vi "Trial v2.vi"(2 "error in (no error)":errorcluster, 3 "queue in":refnum<queue>, 4 "DDA":bool=TRUE) -> (0 "error out":errorcluster, 1 "queue out":refnum<queue>)   [LabVIEW 2017]
uses:
  SubVI/Global.vi
  <vilib>/Analysis/NI_AALPro.lvlib
  <vilib>/robotics/Kinematics/NI_Kinematics.lvlib
  Control/RPY.ctl
  Control/Damping.ctl
  <vilib>/Analysis/NI_AALBase.lvlib
  <vilib>/Analysis/baseanly.llb/Real Dot Product.vi
  <vilib>/Analysis/_algsub.llb/Real Vector Norm.vi
panel:
  in  "Algorithm Parameter":T1={"lambda w"=0.99, "lambda theta"=0.99, "alpha w"=0.01, "alpha theta"=0.01, "alpha Rbar"=0.01}
  in  "n":i32=2
  in  "Reward Parameter":cluster{"C":dbl, "alpha":dbl}={"C"=10.0, "alpha"=1.0}
  in  "lower limit (RoM)":dbl=15.0
  in  "upper limit (RoM)":dbl=85.0
  in  "Time Target (s)":dbl=5.0
  in  "epsilon":dbl=0.1
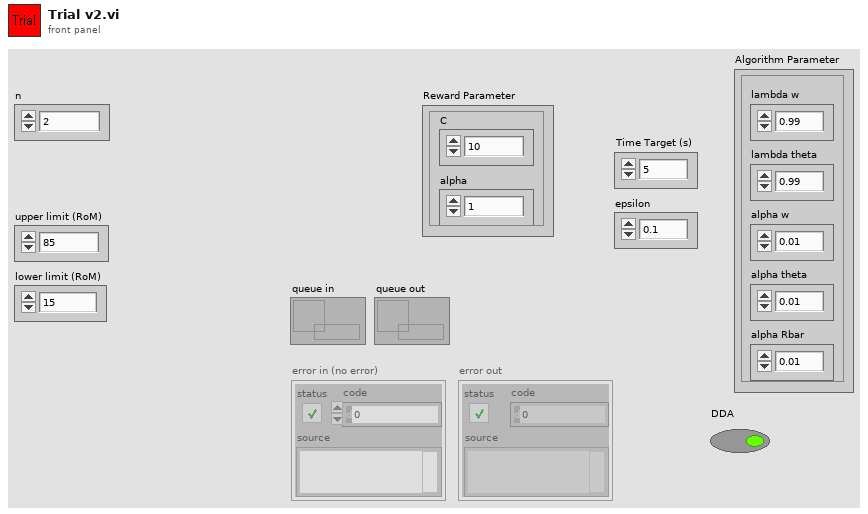
[diagram p1: front panel]
types:
  T1 = cluster{"lambda w":dbl, "lambda theta":dbl, "alpha w":dbl, "alpha theta":dbl, "alpha Rbar":dbl}
  T2 = typedef "Damping.ctl" = cluster{"Cx":dbl, "Cy":dbl, "Cz":dbl}
  T3 = typedef "RPY.ctl" = cluster{"roll":dbl, "pitch":dbl, "yaw":dbl}
  T4 = typedef "NI_Matrix.lvlib/RealMatrix.ctl" = dbl[][]
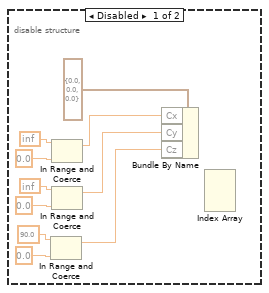
[diagram p2: hidden frame]
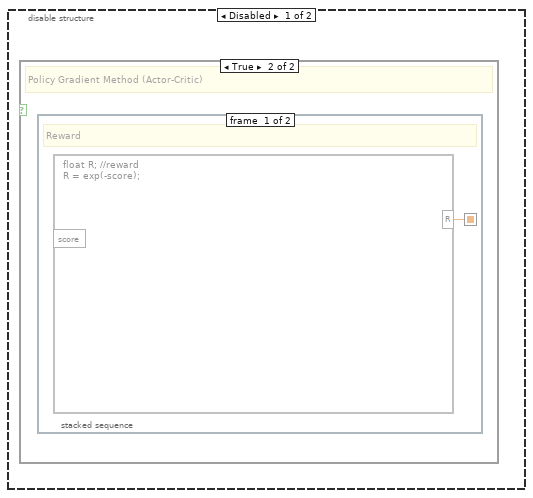
[diagram p3: hidden frame]
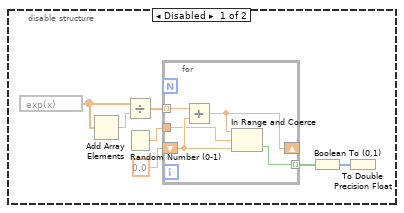
[diagram p6: hidden frame]
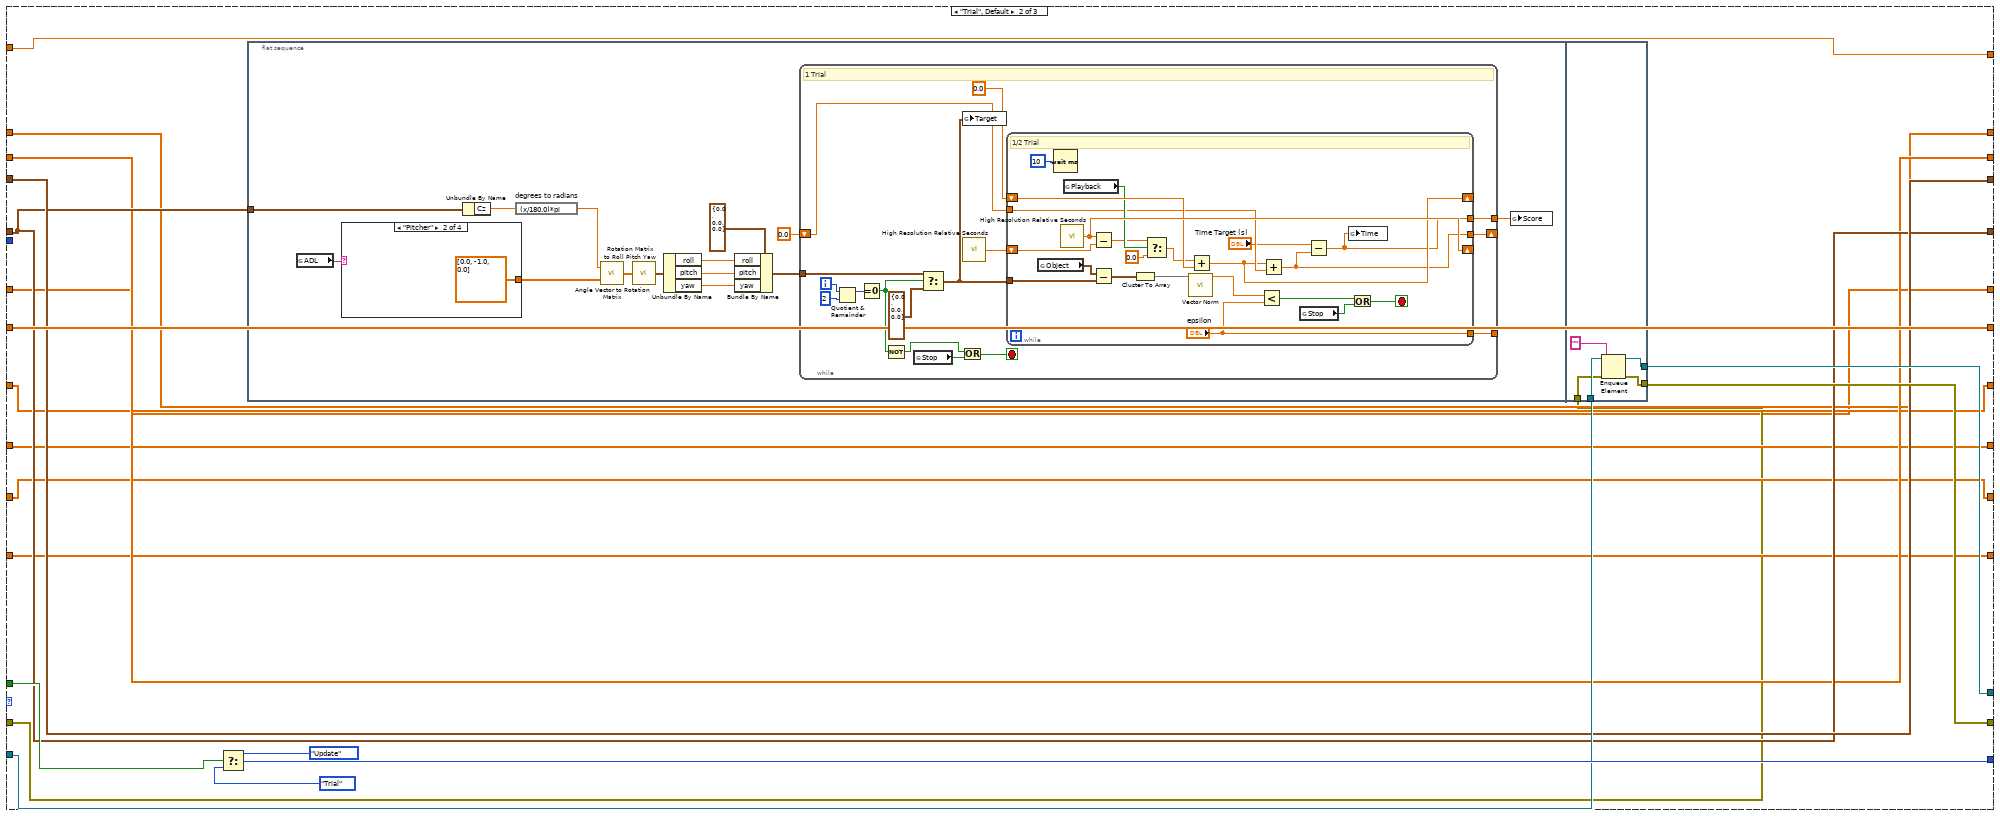
[diagram p7: hidden frame]
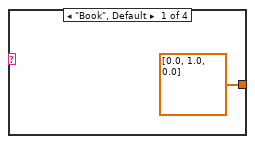
[diagram p8: hidden frame]
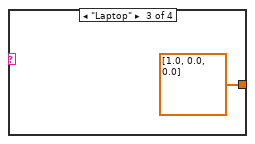
[diagram p9: hidden frame]
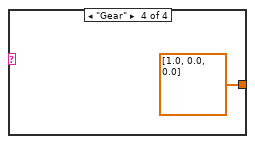
[diagram p10: hidden frame]
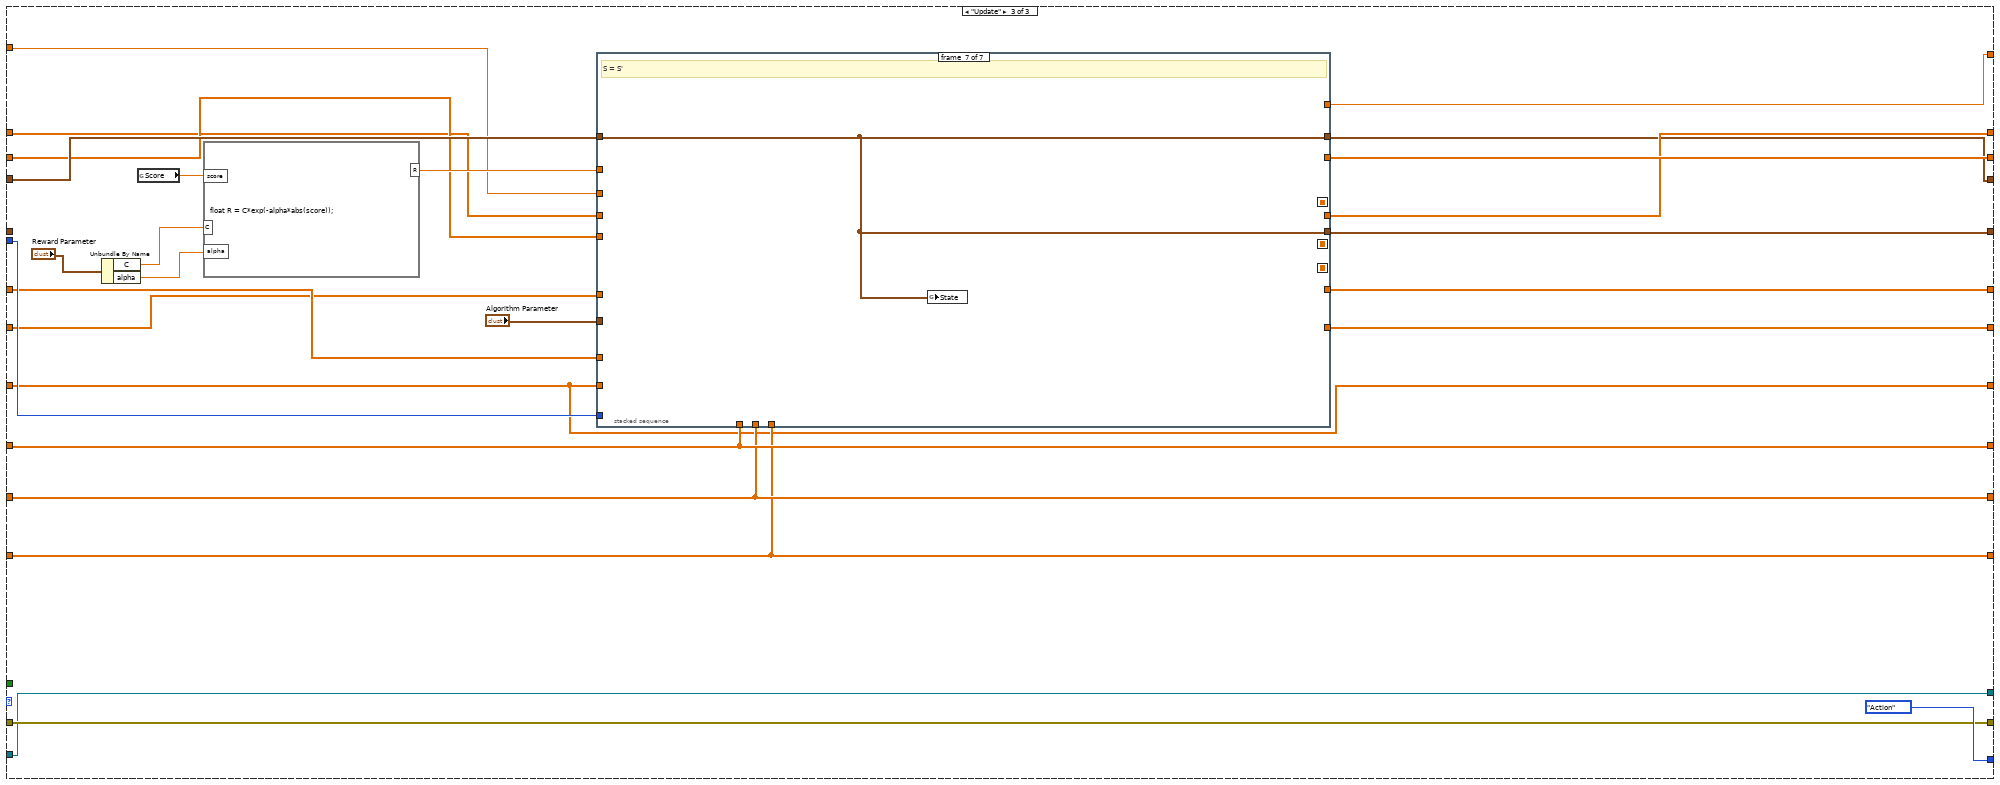
[diagram p11: hidden frame]
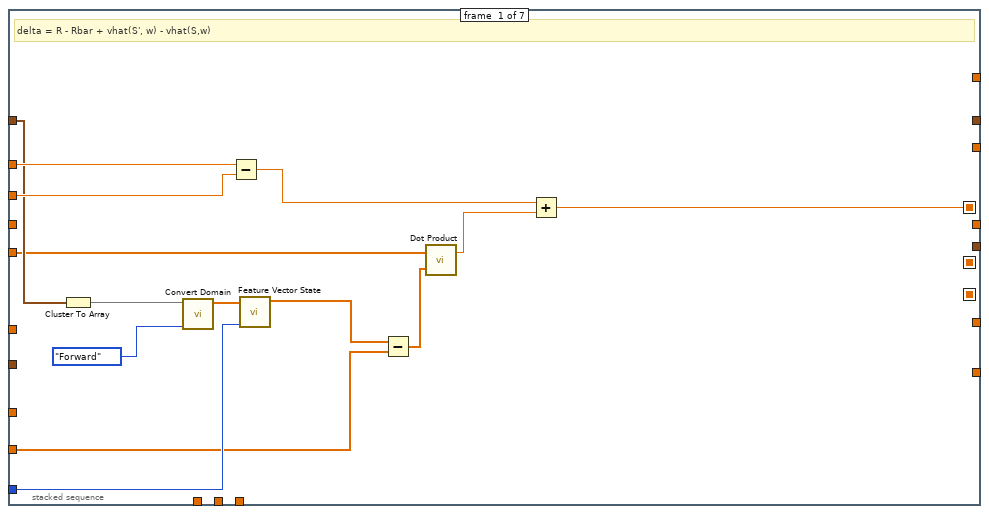
[diagram p12: hidden frame]
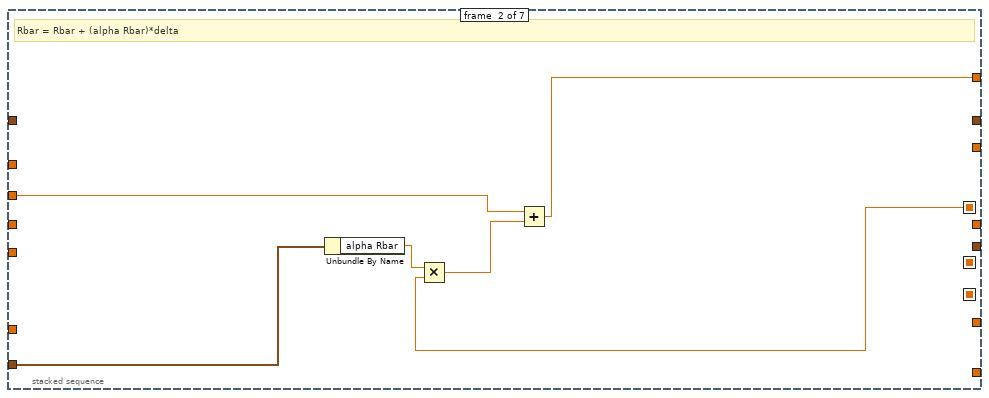
[diagram p13: hidden frame]
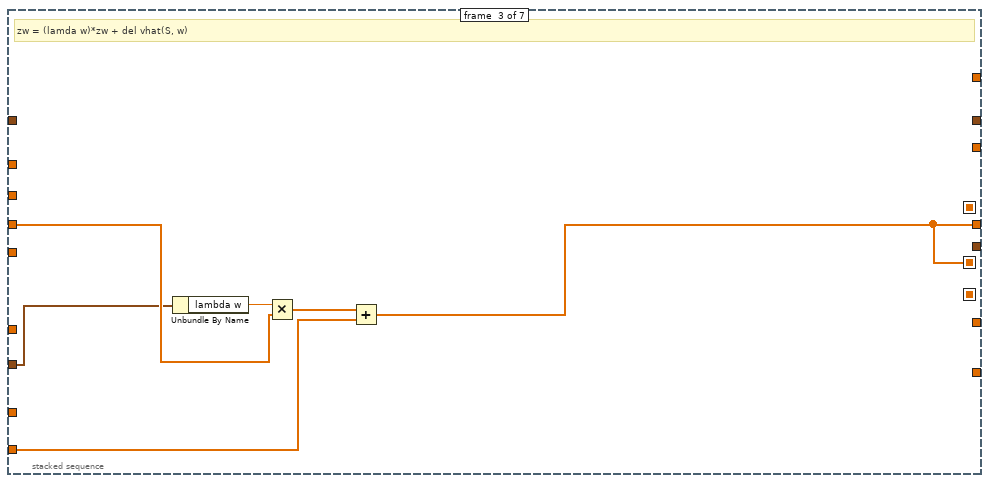
[diagram p14: hidden frame]
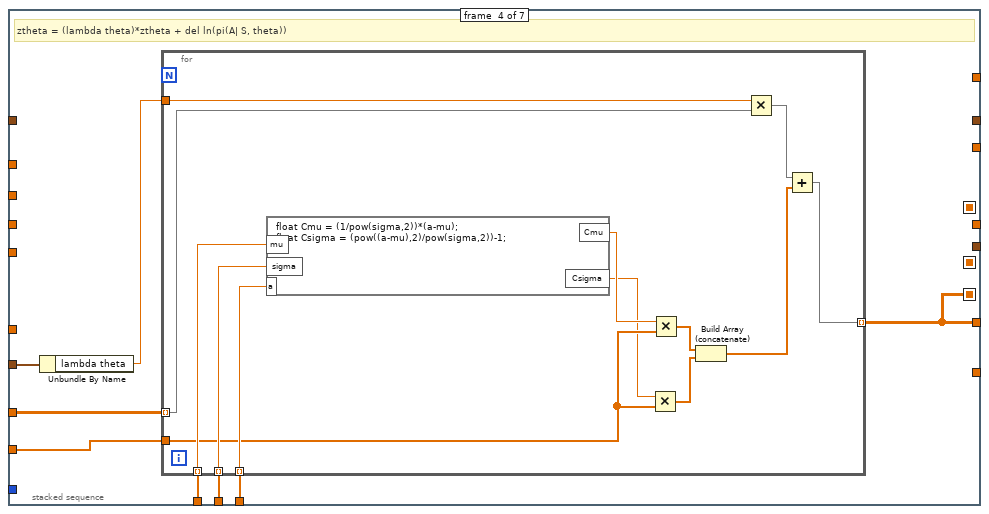
[diagram p15: hidden frame]
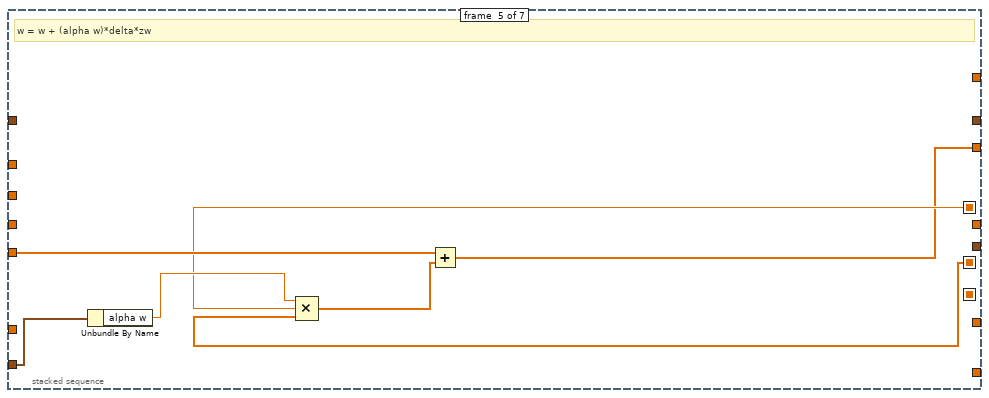
[diagram p16: hidden frame]
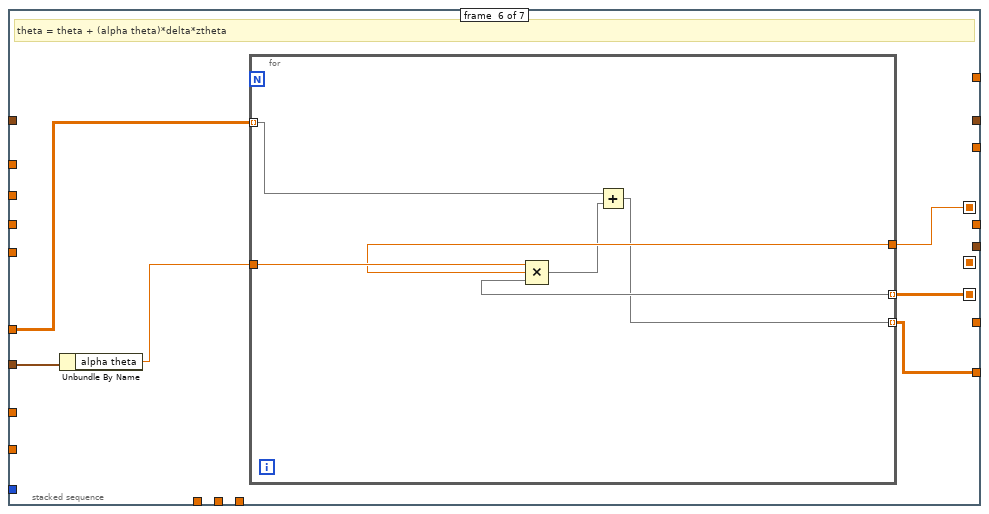
[diagram p17: hidden frame]
diagram:
  n1 = flat-sequence {
    tunnel: "error in (no error)" -> [w23]
    tunnel: "queue in" -> [w25]
    tunnel: "DDA" -> [w18]
    tunnel: [w24] -> w2
    tunnel: [w22] -> w1
    frame #0 {
      n2 = flat-sequence {
        tunnel: ["n"] -> w17
        tunnel: [w38] -> w16
        tunnel: [w37] -> w15
        tunnel: [w37] -> w14
        tunnel: [w31] -> w13
        tunnel: [w29] -> w12
        tunnel: [w29] -> w11
        tunnel: [w31] -> w10
        tunnel: [w29] -> w9
        tunnel: [dbl[] [0.0, 0.0, 0.0]] -> w8
        tunnel: [dbl[] [1.0, 1.0, 1.0]] -> w7
        tunnel: [dbl[] [0.0, 0.0, 0.0]] -> w6
        frame #0 {
          w38 = 0.0  # Rbar
          n3 = call "Feature Vector State.vi"("n x(s)"="n", "state"=dbl[] [0.0, 0.0, 0.0] ("array")) -> ("x(s)"=w34:dbl[])  [unwired: 9 in]
          n4 = Array Size(array=w34) -> (size(s)=w33:i32)
          n5 = Initialize Array(0.0, w33) -> (w29:dbl[])
          n6 = global read "Global.vi" "State"() -> (w37:T2)
          n7 = Build Array (concatenate)(w29, w29) -> (w36:dbl[])
          n8 = Build Array(w36, w36, w36) -> (w31:dbl[][])
        }
      }
      n9 = Select(t=enum16{"Action", "Trial", "Update"}."Action", s=w18, f=enum16{"Action", "Trial", "Update"}."Trial") -> (s? t:f=w19:enum16{"Action", "Trial", "Update"})
      n10 = while {
        shift-right: [w63] -> w24
        shift-left: w25 -> [w65]
        shift-right: [w62] -> w22
        shift-left: w23 -> [w64]
        shift-right: [w67] -> _
        shift-left: w19 -> [w68]
        tunnel: w18 -> [w66]
        tunnel: w17 -> [w61]
        shift-right: [w60] -> _
        shift-left: w13 -> [w59]
        shift-right: [w57] -> _
        shift-left: w16 -> [w58]
        shift-right: [w53] -> _
        shift-left: w15 -> [w55]
        shift-right: [w56] -> _
        shift-left: w14 -> [w54]
        shift-right: [w51] -> _
        shift-left: w12 -> [w52]
        shift-right: [w49] -> _
        shift-left: w11 -> [w50]
        shift-right: [w39] -> _
        shift-left: w10 -> [w48]
        shift-right: [w47] -> _
        shift-left: w9 -> [w46]
        shift-right: [w45] -> _
        shift-left: w8 -> [w44]
        shift-right: [w42] -> _
        shift-left: w7 -> [w43]
        shift-right: [w40] -> _
        shift-left: w6 -> [w41]
        stop <- w69 stop-if-true
        # "State Machine"
        n11 = case shown="\"Action\"" w68 {
          tunnel: [enum16{"Action", "Trial", "Update"}."Trial" w129 enum16{"Action", "Trial", "Update"}."Action"] -> w67
          tunnel: w66 -> [_ w131 _]
          tunnel: w65 -> [w84 w128 w217]
          tunnel: w64 -> [w85 w114 w218]
          tunnel: [w84 w127 w217] -> w63
          tunnel: [w85 w126 w218] -> w62
          tunnel: w61 -> [w77 _ w208]
          tunnel: [w83 w124 w196] -> w60
          tunnel: w59 -> [w83 w124 w198]
          tunnel: w58 -> [w80 w123 w210]
          tunnel: [w80 w123 w206] -> w57
          tunnel: w55 -> [w78 w121 _]
          tunnel: [w79 w122 w195] -> w56
          tunnel: w54 -> [_ w122 w212]
          tunnel: [w78 w121 w194] -> w53
          tunnel: w52 -> [w76 w120 w209]
          tunnel: [w76 w120 w205] -> w51
          tunnel: w50 -> [w75 w119 w204]
          tunnel: [w75 w119 w203] -> w49
          tunnel: w48 -> [w70 w113 w202]
          tunnel: [w74 w118 w193] -> w47
          tunnel: w46 -> [_ w118 w193]
          tunnel: [w73 w117 w201] -> w45
          tunnel: w44 -> [_ w117 w201]
          tunnel: w43 -> [_ w116 w200]
          tunnel: [w72 w116 w200] -> w42
          tunnel: w41 -> [_ w115 w199]
          tunnel: [w71 w115 w199] -> w40
          tunnel: [w70 w113 w197] -> w39
          frame "Action" {
            n12 = Cluster To Array(cluster=w78) -> (array=w81:dbl[])
            n13 = call "Convert Domain.vi"("Direction"=enum16{"Forward", "Backward"}."Forward", "Real"=w81) -> ("Unit"=w86:dbl[])  [unwired: 9 in]
            n14 = call "Feature Vector State.vi"("n x(s)"=w77, "state"=w86) -> ("x(s)"=w74:dbl[])  [unwired: 9 in]
            n15 = Array Size(array=w74) -> (size(s)=w82:i32)
            n16 = for {
              tunnel: w83 -> [w112] mode=indexing
              tunnel: w74 -> [w109]
              tunnel: w74 -> [w108]
              tunnel: [w106] -> w71 mode=indexing
              tunnel: w82 -> [w105]
              tunnel: [w104] -> w73 mode=indexing
              tunnel: [w103] -> w72 mode=indexing
              n17 = Split 1D Array(array=w112, index=w105) -> (first subarray=w111:dbl[], second subarray=w110:dbl[])
              n18 = call-poly <vilib>:"Dot Product.vi"("Y Vector"=w108, "X Vector"=w110) -> ("X * Y"=w107:dbl)  [unwired: 1 out]
              n19 = call-poly <vilib>:"Dot Product.vi"("Y Vector"=w109, "X Vector"=w111) -> ("X * Y"=w104:dbl)  [unwired: 1 out]
              n20 = Exponential(1:w107) -> (0:w103:dbl)
              n21 = call "Box-Muller.vi"("sigma"=w103, "mu"=w104) -> ("x"=w106:dbl)  [unwired: 9 in]
            }
            n22 = flat-sequence {
              tunnel: w71 -> [w102]
              tunnel: w81 -> [w98]
              tunnel: [w89] -> w79
              frame #0 {
                # "Observe S' in Real Domain"
                n23 = Multiply(x=0.1, y=w102) -> (x*y=w100:dbl[])
                n24 = Increment(x=w100) -> (x+1=w99:dbl[])
                n25 = Multiply(x=w99, y=w98) -> (x*y=w94:dbl[])
                n26 = Index Array(array=w94) -> (element #1=w96:dbl, element #2=w95:dbl, element #3=w93:dbl)  [unwired: 3 in]
                n27 = In Range and Coerce(upper limit="upper limit (RoM)", x=w93, lower limit="lower limit (RoM)") -> (coerced(x)=w92:dbl)  [unwired: 1 out]
                n28 = Bundle By Name(cluster=T2 {"Cx"=0.0, "Cy"=0.0, "Cz"=0.0} ("State"), "Cx"=w96, "Cy"=w95, "Cz"=w92) -> (w89:T2)
              }
            }
          }
          frame "Trial", Default {
            n29 = Select(t=enum16{"Action", "Trial", "Update"}."Update", s=w131, f=enum16{"Action", "Trial", "Update"}."Trial") -> (s? t:f=w129:enum16{"Action", "Trial", "Update"})
            n30 = flat-sequence {
              tunnel: w121 -> [w132]
              tunnel: w128 -> [w192]
              tunnel: [w191] -> w127
              tunnel: [w190] -> w126
              tunnel: w114 -> [w188]
              frame #0 {
                n31 = global read "Global.vi" "ADL"() -> (w136:string)
                n32 = case shown="\"Pitcher\"" w136 {
                  tunnel: [dbl[] [0.0, 1.0, 0.0] dbl[] [0.0, -1.0, 0.0] dbl[] [1.0, 0.0, 0.0] dbl[] [1.0, 0.0, 0.0]] -> w135
                  frame "Book", Default {
                  }
                  frame "Pitcher" {
                  }
                  frame "Laptop" {
                  }
                  frame "Gear" {
                  }
                }
                n33 = Unbundle By Name(w132) -> ("Cz"=w134:dbl)
                n34 = expression code="(x/180.0)*pi" "degrees to radians"(w134) -> (w137:dbl)
                n35 = call <vilib>:"Angle Vector to Rotation Matrix.vi"("vector"=w135, "angle"=w137) -> ("rotation matrix"=w140:T4)
                n36 = call <vilib>:"Rotation Matrix to Roll Pitch Yaw.vi"("rotation matrix"=w140) -> ("angles"=w141:cluster{"roll":dbl, "pitch":dbl, "yaw":dbl})
                n37 = Unbundle By Name(w141) -> ("roll"=w142:dbl, "pitch"=w143:dbl, "yaw"=w144:dbl)
                n38 = Bundle By Name(cluster=T3 {"roll"=0.0, "pitch"=0.0, "yaw"=0.0} ("Target"), "roll"=w142, "pitch"=w143, "yaw"=w144) -> (w138:T3)
                n39 = while {
                  tunnel: w138 -> [w160]
                  shift-right: [w152] -> _
                  shift-left: 0.0 -> [w153]
                  tunnel: [w151] -> _
                  tunnel: [w150] -> w133
                  i -> [w163]
                  stop <- w156 stop-if-true
                  # "1 Trial"
                  n40 = Quotient & Remainder(x=w163, y=2) -> (x-y*floor(x/y)=w161:i32)  [unwired: 1 out]
                  n41 = Equal To 0?(x=w161) -> (x = 0?=w155:bool)
                  n42 = Not(x=w155) -> (.not. x?=w154:bool)
                  n43 = global read "Global.vi" "Stop"() -> (w157:bool)
                  n44 = Select(t=w160, s=w155, f=T3 {"roll"=0.0, "pitch"=0.0, "yaw"=0.0} ("Target")) -> (s? t:f=w158:T3)
                  n45 = Or(x=w154, y=w157) -> (x .or. y?=w156:bool)
                  n46 = global write "Global.vi" "Target"(w158) -> ()
                  n47 = call <vilib>:"High Resolution Relative Seconds.vi"() -> ("relative seconds"=w165:dbl)
                  n48 = while {
                    tunnel: w158 -> [w172]
                    shift-right: [w178] -> _
                    shift-left: w165 -> [w179]
                    shift-right: [w170] -> _
                    shift-left: 0.0 -> [w177]
                    tunnel: w153 -> [w171]
                    tunnel: [w168] -> w152
                    tunnel: ["epsilon"] -> w151
                    tunnel: [w166] -> w150
                    stop <- w180 stop-if-true
                    # "1/2 Trial"
                    n49 = global read "Global.vi" "Object"() -> (w185:T3)
                    n50 = Wait (ms)(milliseconds to wait=u32 10) -> ()  [unwired: 1 out]
                    n51 = call <vilib>:"High Resolution Relative Seconds.vi"() -> ("relative seconds"=w178:dbl)
                    n52 = global read "Global.vi" "Playback"() -> (w176:bool)
                    n53 = Subtract(x=w178, y=w179) -> (x-y=w175:dbl)
                    n54 = Subtract(x=w185, y=w172) -> (x-y=w186:T3)
                    n55 = Cluster To Array(cluster=w186) -> (array=w187:dbl[])
                    n56 = Select(t=w175, s=w176, f=0.0) -> (s? t:f=w174:dbl)
                    n57 = call-poly <vilib>:"Vector Norm.vi"("Input Vector"=w187) -> ("norm"=w184:dbl)  [unwired: 9 in, 1 out]
                    n58 = Add(x=w174, y=w177) -> (x+y=w170:dbl)
                    n59 = Less?(x=w184, y="epsilon") -> (x < y?=w183:bool)
                    n60 = Add(x=w170, y=w171) -> (x+y=w168:dbl)
                    n61 = global read "Global.vi" "Stop"() -> (w182:bool)
                    n62 = Subtract(x="Time Target (s)", y=w168) -> (x-y=w166:dbl)
                    n63 = global write "Global.vi" "Time"(w166) -> ()
                    n64 = Or(x=w183, y=w182) -> (x .or. y?=w180:bool)
                  }
                }
                n65 = global write "Global.vi" "Score"(w133) -> ()
              }
              frame #1 {
                n66 = Enqueue Element(queue=w192, element="", error in (no error)=w188) -> (queue out=w191:refnum<queue>, error out=w190:errorcluster)  [unwired: 1 in, 1 out]
              }
            }
          }
          frame "Update" {
            n67 = Unbundle By Name("Reward Parameter") -> ("C"=w214:dbl, "alpha"=w213:dbl)
            n68 = global read "Global.vi" "Score"() -> (w216:dbl)
            n69 = formula code="float R = C*exp(-alpha*abs(score));"("score"=w216, "C"=w214, "alpha"=w213) -> ("R"=w211:dbl)
            n70 = stacked-sequence {
              seq-local: [w229 _ _ _ _ _ _] -> [_ w236 _ _ w270 w276 _]
              seq-local: [_ _ w240 _ _ _ _] -> [_ _ _ _ w269 _ _]
              seq-local: [_ _ _ w246 _ _ _] -> [_ _ _ _ _ w275 _]
              tunnel: w212 -> [w228 _ _ _ _ _ w286]
              tunnel: w211 -> [w233 _ _ _ _ _ _]
              tunnel: w210 -> [w232 w239 _ _ _ _ _]
              tunnel: w209 -> [w224 _ _ _ w273 _ _]
              tunnel: w208 -> [w226 _ _ _ _ _ _]
              tunnel: "Algorithm Parameter" -> [_ w238 w244 w252 w272 w279 _]
              tunnel: [_ w234 _ _ _ _ _] -> w206
              tunnel: [_ _ _ _ w268 _ _] -> w205
              tunnel: w204 -> [_ _ w245 _ _ _ _]
              tunnel: [_ _ w240 _ _ _ _] -> w203
              tunnel: w202 -> [_ _ _ w253 _ _ _]
              tunnel: w193 -> [w221 _ w241 w247 _ _ _]
              tunnel: w201 -> [_ _ _ w250 _ _ _]
              tunnel: w200 -> [_ _ _ w249 _ _ _]
              tunnel: w199 -> [_ _ _ w248 _ _ _]
              tunnel: w198 -> [_ _ _ _ _ w278 _]
              tunnel: [_ _ _ w246 _ _ _] -> w197
              tunnel: [_ _ _ _ _ w274 _] -> w196
              tunnel: [_ _ _ _ _ _ w286] -> w195
              tunnel: [_ _ _ _ _ _ w286] -> w194
              frame #0 {
                # "delta = R - Rbar + vhat(S', w) - vhat(S,w)"
                n71 = Cluster To Array(cluster=w228) -> (array=w227:dbl[])
                n72 = call "Convert Domain.vi"("Direction"=enum16{"Forward", "Backward"}."Forward", "Real"=w227) -> ("Unit"=w230:dbl[])  [unwired: 9 in]
                n73 = Subtract(x=w233, y=w232) -> (x-y=w231:dbl)
                n74 = call "Feature Vector State.vi"("n x(s)"=w226, "state"=w230) -> ("x(s)"=w222:dbl[])  [unwired: 9 in]
                n75 = Subtract(x=w222, y=w221) -> (x-y=w220:dbl[])
                n76 = call-poly <vilib>:"Dot Product.vi"("Y Vector"=w220, "X Vector"=w224) -> ("X * Y"=w223:dbl)  [unwired: 1 out]
                n77 = Add(x=w231, y=w223) -> (x+y=w229:dbl)
              }
              frame #1 {
                # "Rbar = Rbar + (alpha Rbar)*delta"
                n78 = Unbundle By Name(w238) -> ("alpha Rbar"=w237:dbl)
                n79 = Multiply(x=w237, y=w236) -> (x*y=w235:dbl)
                n80 = Add(x=w239, y=w235) -> (x+y=w234:dbl)
              }
              frame #2 {
                # "zw = (lamda w)*zw + del vhat(S, w)"
                n81 = Unbundle By Name(w244) -> ("lambda w"=w243:dbl)
                n82 = Multiply(x=w243, y=w245) -> (x*y=w242:dbl[])
                n83 = Add(x=w242, y=w241) -> (x+y=w240:dbl[])
              }
              frame #3 {
                # "ztheta = (lambda theta)*ztheta + del ln(pi(A| S, theta))"
                n84 = Unbundle By Name(w252) -> ("lambda theta"=w251:dbl)
                n85 = for {
                  tunnel: w253 -> [w265] mode=indexing
                  tunnel: w251 -> [w266]
                  tunnel: w250 -> [w264] mode=indexing
                  tunnel: w249 -> [w263] mode=indexing
                  tunnel: w248 -> [w262] mode=indexing
                  tunnel: w247 -> [w260]
                  tunnel: [w254] -> w246 mode=indexing
                  n86 = formula code="float Cmu = (1/pow(sigma,2))*(a-mu);\nfloat Csigma = (pow((a-mu),2)/pow(sigma,2))-1;"("mu"=w264, "sigma"=w263, "a"=w262) -> ("Cmu"=w261:dbl, "Csigma"=w259:dbl)
                  n87 = Multiply(x=w259, y=w260) -> (x*y=w257:dbl[])
                  n88 = Multiply(x=w261, y=w260) -> (x*y=w258:dbl[])
                  n89 = Build Array (concatenate)(w258, w257) -> (w255:dbl[])
                  n90 = Multiply(x=w266, y=w265) -> (x*y=w256:dbl[])
                  n91 = Add(x=w256, y=w255) -> (x+y=w254:dbl[])
                }
              }
              frame #4 {
                # "w = w + (alpha w)*delta*zw"
                n92 = Unbundle By Name(w272) -> ("alpha w"=w271:dbl)
                n93 = Compound Arithmetic op=MULTIPLY(w271, w270, w269) -> (w267:dbl[])
                n94 = Add(x=w273, y=w267) -> (x+y=w268:dbl[])
              }
              frame #5 {
                # "theta = theta + (alpha theta)*delta*ztheta"
                n95 = Unbundle By Name(w279) -> ("alpha theta"=w277:dbl)
                n96 = for {
                  tunnel: w278 -> [w285] mode=indexing
                  tunnel: w277 -> [w284]
                  tunnel: w276 -> [w283]
                  tunnel: w275 -> [w282] mode=indexing
                  tunnel: [w280] -> w274 mode=indexing
                  n97 = Compound Arithmetic op=MULTIPLY(w284, w283, w282) -> (w281:dbl[])
                  n98 = Add(x=w285, y=w281) -> (x+y=w280:dbl[])
                }
              }
              frame #6 {
                # "S = S'"
                n99 = global write "Global.vi" "State"(w286) -> ()
              }
            }
          }
        }
        n100 = global read "Global.vi" "Stop"() -> (w69:bool)
      }
    }
  }
  n101 = disable-structure shown="Enabled" {
    frame Disabled {
      n102 = In Range and Coerce(upper limit=90.0, lower limit=0.0) -> (coerced(x)=w296:dbl)  [unwired: 1 in, 1 out]
      n103 = In Range and Coerce(upper limit=inf, lower limit=0.0) -> (coerced(x)=w294:dbl)  [unwired: 1 in, 1 out]
      n104 = In Range and Coerce(upper limit=inf, lower limit=0.0) -> (coerced(x)=w295:dbl)  [unwired: 1 in, 1 out]
      n105 = Bundle By Name(cluster=T2 {"Cx"=0.0, "Cy"=0.0, "Cz"=0.0} ("State"), "Cx"=w294, "Cy"=w295, "Cz"=w296) -> ()  [unwired: 1 out]
      n106 = Index Array() -> ()  [unwired: 4 in, 3 out]
    }
    frame Enabled {
    }
  }
  n107 = disable-structure shown="Enabled" {
    frame Disabled {
      n108 = expression code="exp(x)"() -> (w299:dbl[])  [unwired: 1 in]
      n109 = Add Array Elements(numeric array=w299) -> (sum=w300:dbl)
      n110 = Divide(x=w299, y=w300) -> (x/y=w297:dbl[])
      n111 = Random Number (0-1)() -> (number: 0 to 1=w301:dbl)
      n112 = for {
        shift-right: [w307] -> _
        shift-left: 0.0 -> [w308]
        tunnel: w301 -> [w306]
        tunnel: [w305] -> w302 mode=indexing
        tunnel: w297 -> [w304] mode=indexing
        n113 = Add(x=w304, y=w308) -> (x+y=w307:dbl)
        n114 = In Range and Coerce(upper limit=w307, x=w306, lower limit=w308) -> (In Range?=w305:bool)  [unwired: 1 out]
      }
      n115 = Boolean To (0,1)(Boolean=w302) -> (0, 1=w303:i16[])
      n116 = To Double Precision Float(number=w303) -> ()  [unwired: 1 out]
    }
    frame Enabled {
    }
  }
  n117 = disable-structure shown="Enabled" {
    frame Disabled {
      n118 = case shown="True" {
        selector: _ -> [_ _]
        frame False {
        }
        frame True {
          # "Policy Gradient Method (Actor-Critic)"
          n119 = stacked-sequence {
            seq-local: [w309 _] -> [_ _]
            frame #0 {
              # "Reward"
              n120 = formula code="float R; //reward\nR = exp(-score);"() -> ("R"=w309:dbl)  [unwired: 1 in]
            }
            frame #1 {
            }
          }
        }
      }
    }
    frame Enabled {
    }
  }
  "error out" <- w1
  "queue out" <- w2
